vi "Init Splash.vi"(8 "error in (no error)":errorcluster, 11 "Basic Splash in":refnum<class "Basic Splash.lvclass">) -> (0 "error out":errorcluster, 3 "Basic Splash out":refnum<class "Basic Splash.lvclass">)   [LabVIEW 2020, in "Volatus.lvlib" / "Basic Splash.lvclass"]
uses:
  Basic Splash.lvclass
  Basic Splash.lvclass/Basic Splash.ctl
  Event Type.ctl
  Event Data.ctl
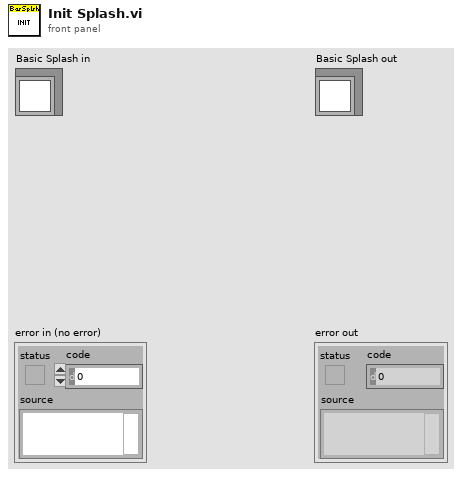
[diagram p1: front panel]
types:
  T1 = typedef "Volatus.lvlib/Basic Splash.lvclass/Event Data.ctl" = cluster{"Type":T2, "Status":string}
  T2 = typedef "Volatus.lvlib/Basic Splash.lvclass/Event Type.ctl" = enum16{"Show", "Hide", "Update", "Close"}
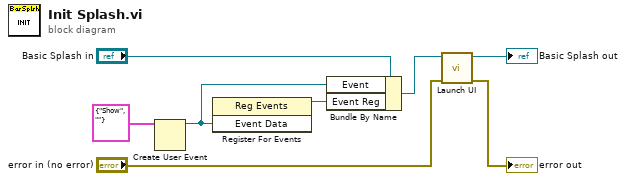
[diagram p0: block diagram]
diagram:
  n1 = Create User Event(user event datatype=T1 {"Type"=enum."Show", "Status"=""} ("Event Data")) -> (user event=w4:refnum<user-event>)  [unwired: 1 in, 1 out]
  n2 = register-events(w4) -> (reference out=w5:refnum<event-registration>)  [unwired: 2 in, 1 out]
  n3 = Bundle By Name(cluster="Basic Splash in", "Event"=w4, "Event Reg"=w5) -> (w6:refnum<class "Basic Splash.lvclass">)
  n4 = call "Launch UI.vi"("error in (no error)"="error in (no error)", "Basic Splash in"=w6) -> ("error out"=→"error out":errorcluster, "Basic Splash out"=→"Basic Splash out":refnum<class "Basic Splash.lvclass">)  [unwired: 8 in]
